vi "PRIOR_v.10.vi"() -> ()   [LabVIEW 2018]
uses:
  <vilib>/Instr/_visa.llb/VISA Configure Serial Port (Instr).vi
panel:
  in  "数字":i32
  in  "VISA resource name":refnum<visa-resource-name> caption="VISA资源名称"
  in  "返回Z轴坐标":bool
  in  "设置移动步长":bool
  in  "停止运动":bool
  out "error out":errorcluster
  out "读取缓冲区":string
  in  "error in (no error)":errorcluster caption="错误输入（无错误）"
  in  "down":bool
  in  "up":bool
  in  "停止":bool
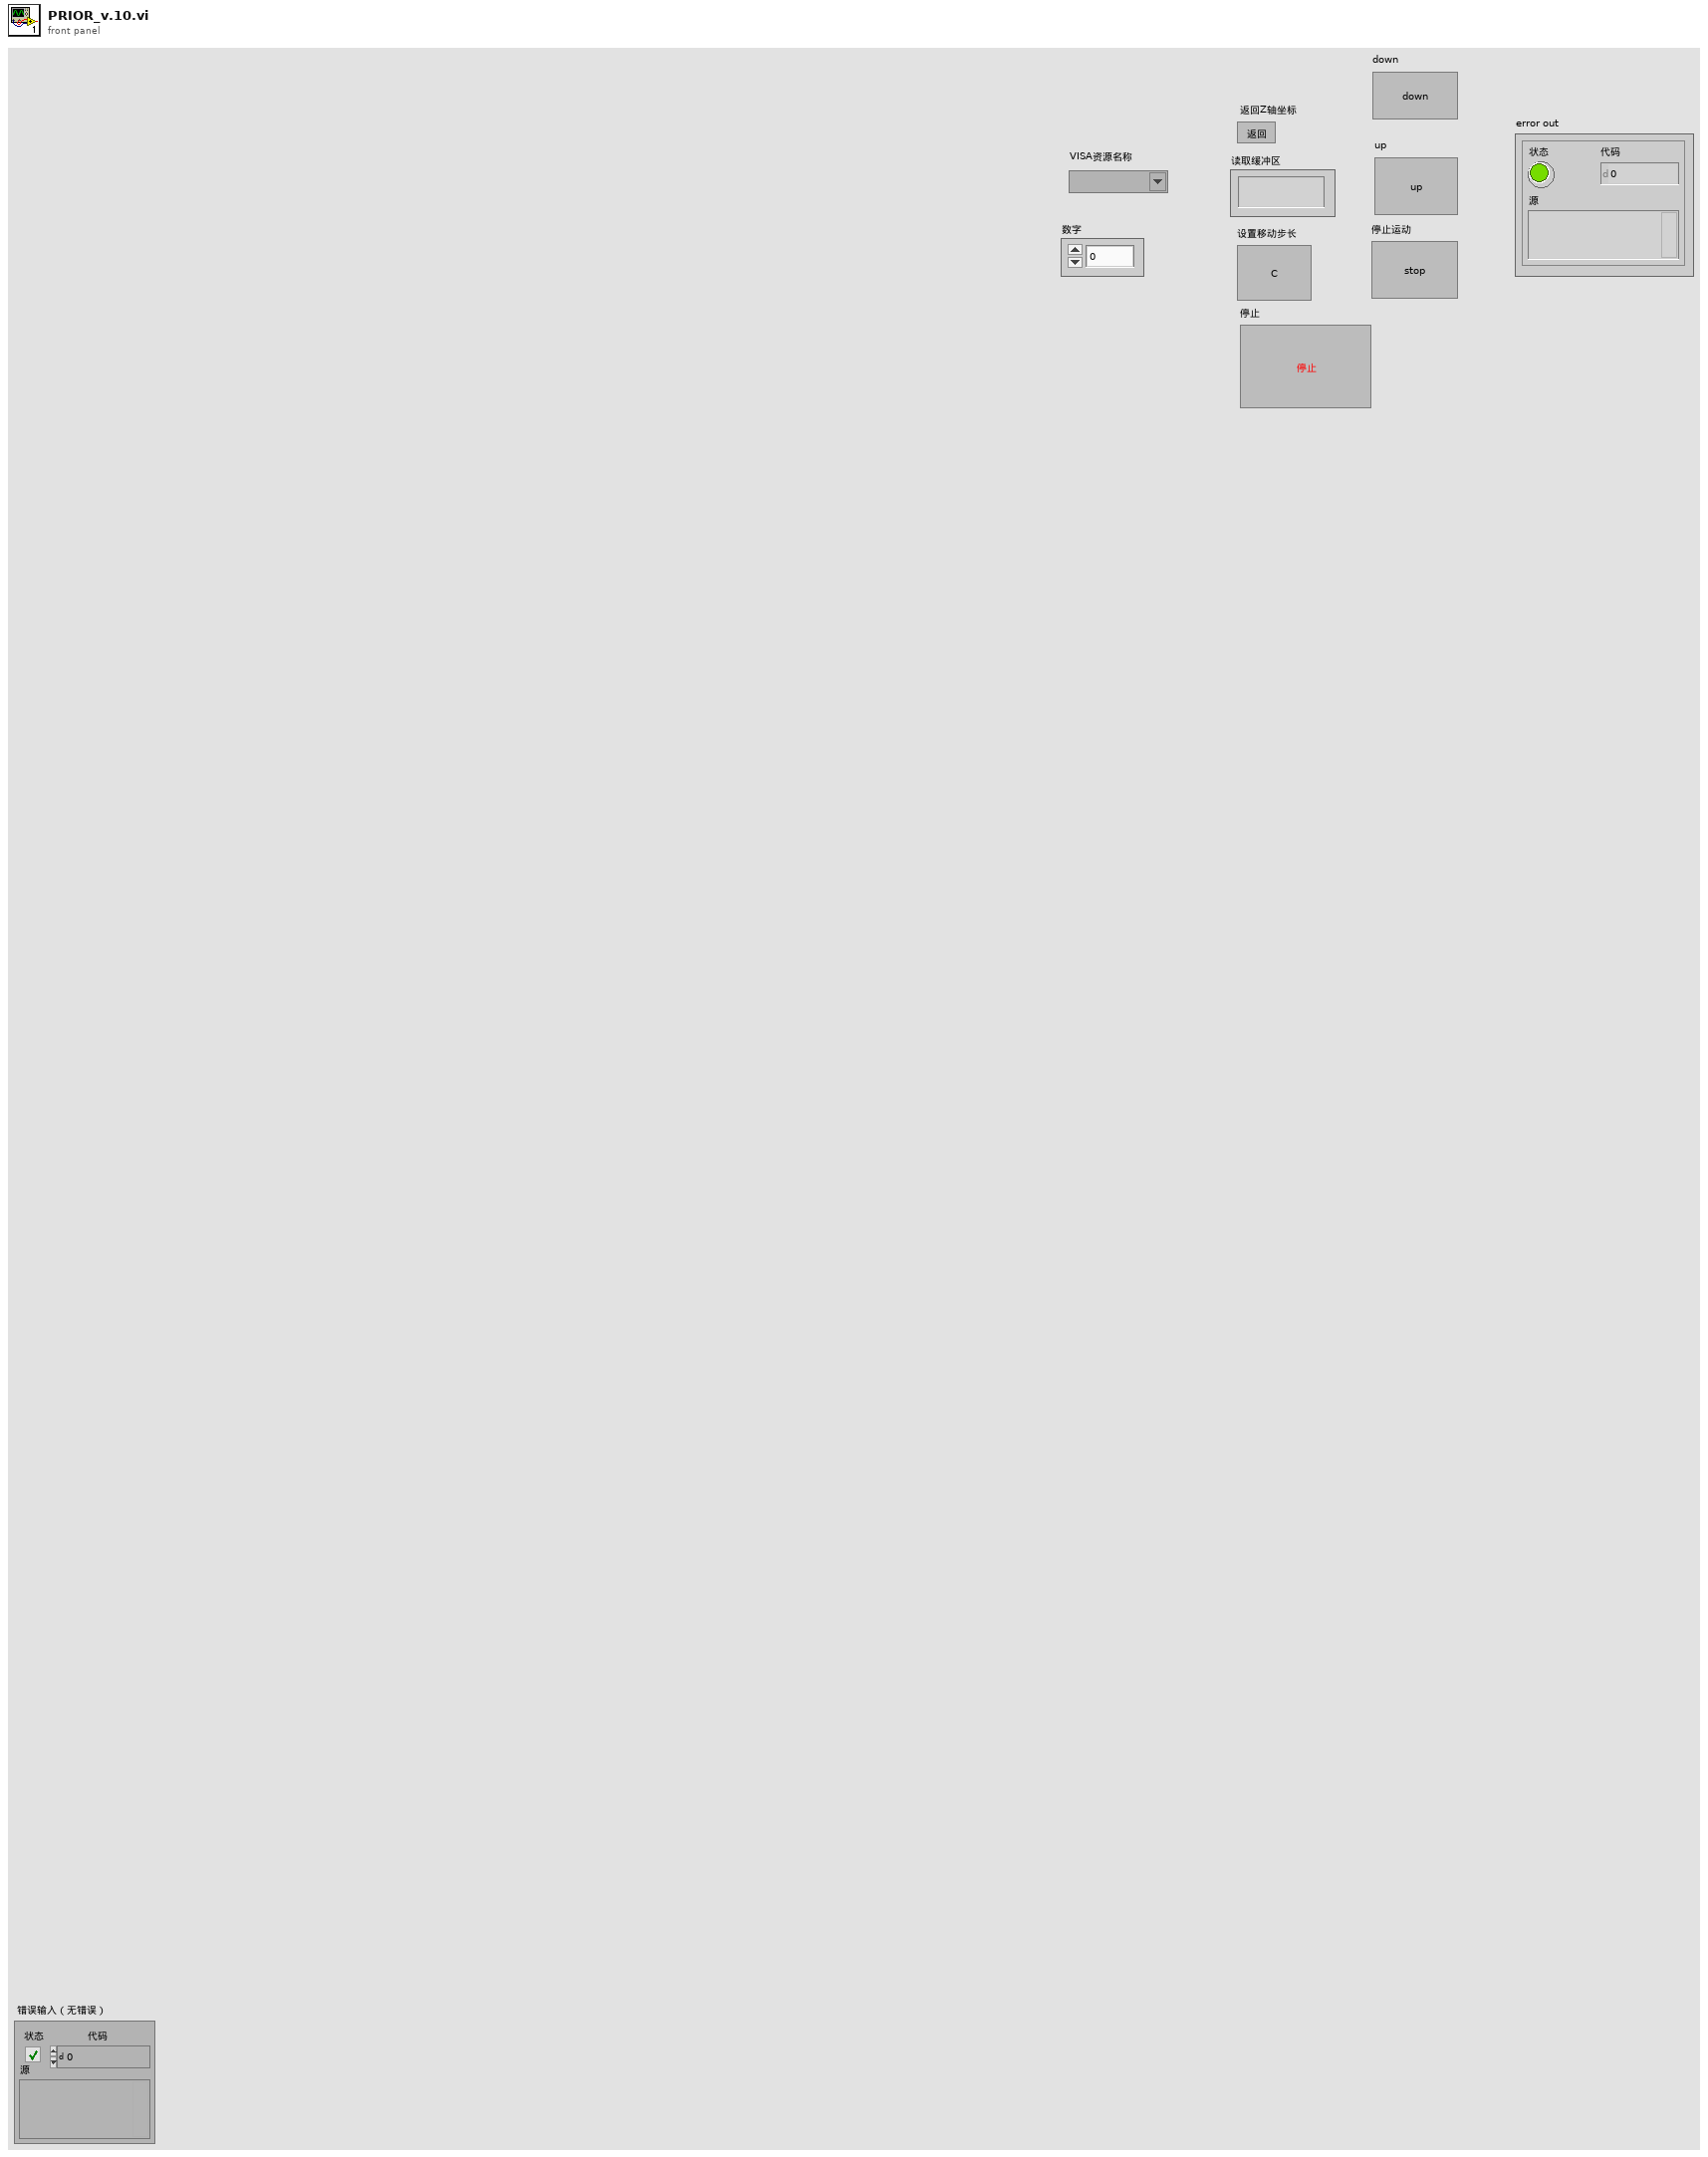
[diagram p1: front panel]
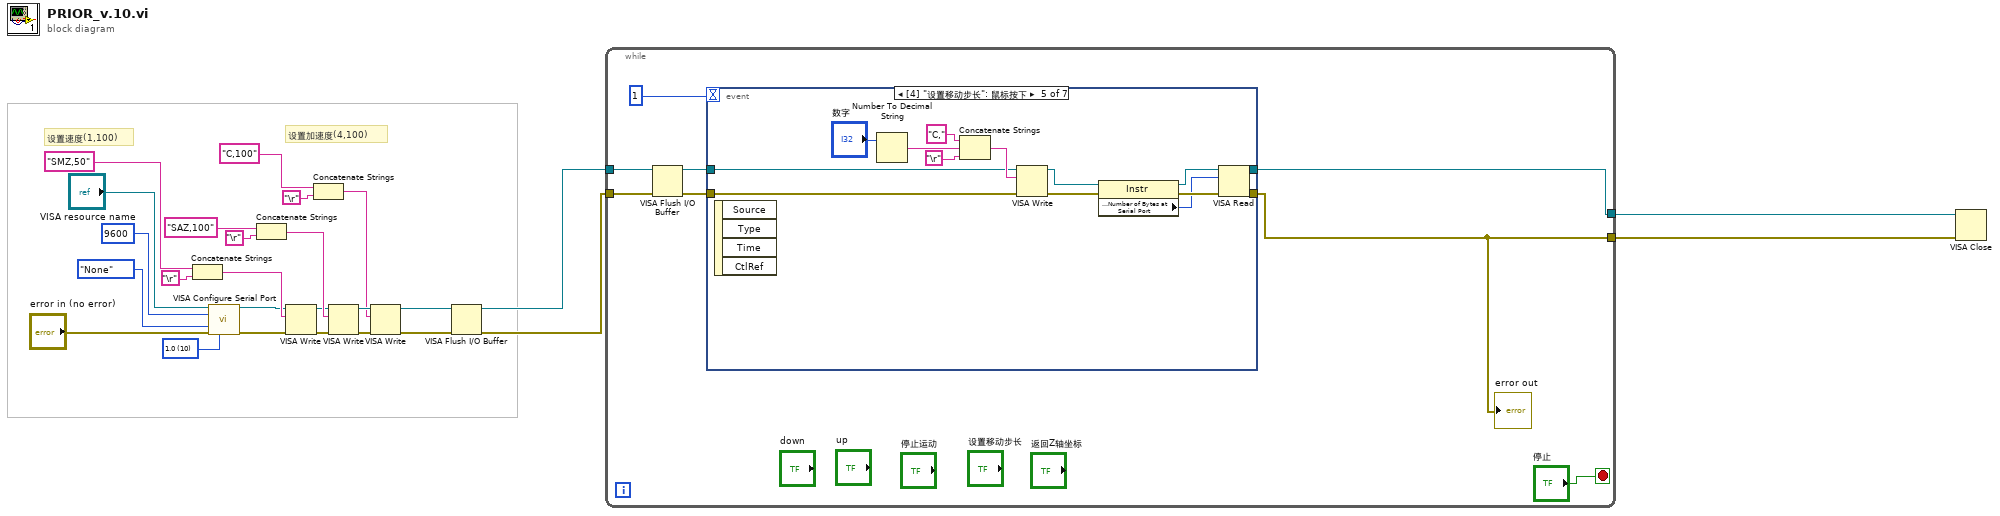
[diagram p0: block diagram]
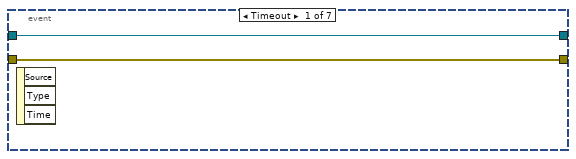
[diagram p2: hidden frame]
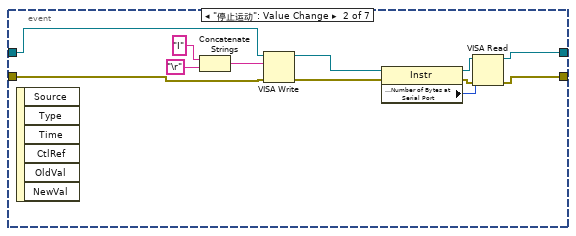
[diagram p3: hidden frame]
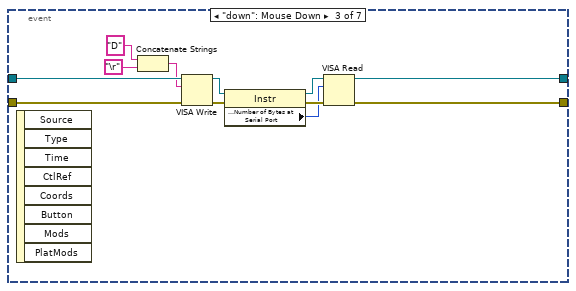
[diagram p4: hidden frame]
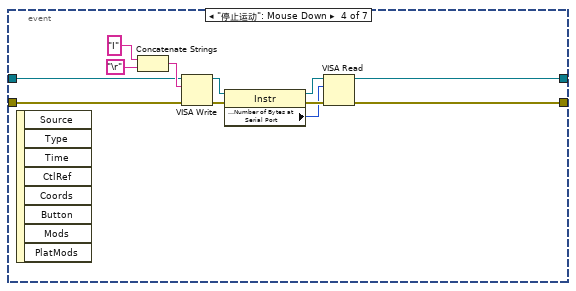
[diagram p5: hidden frame]
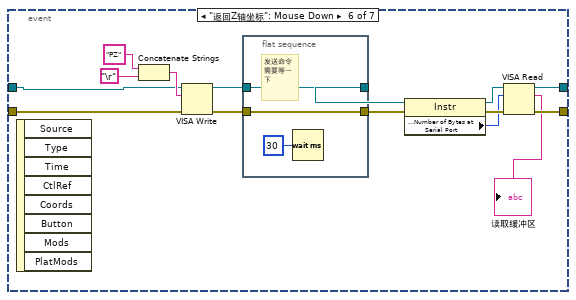
[diagram p6: hidden frame]
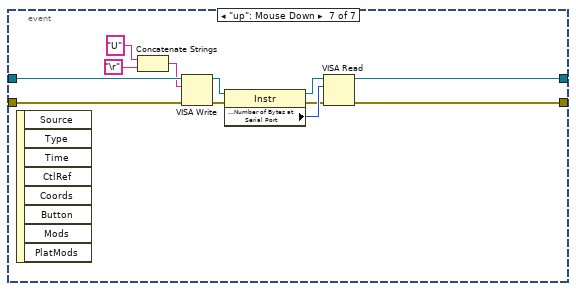
[diagram p7: hidden frame]
diagram:
  w24 = u16 10 items=["1.0"=10, "1.5"=15, "2.0"=20] ("停止位 (10: 1位)")
  # "设置加速度(4,100)"
  # "设置速度(1,100)"
  n1 = Concatenate Strings("SMZ,50" ("写入缓冲区"), "\r") -> (w20:string)
  n2 = call-poly "VISA Configure Serial Port"("VISA resource name"="VISA resource name", "baud rate (9600)"=u32 9600 ("波特率(9600)"), "parity (0:none)"=enum16{"None", "Odd", "Even", "Mark", "Space"}."None" ("校验（无）"), "error in (no error)"="error in (no error)", "stop bits (10: 1 bit)"=w24) -> ("VISA resource name out"=w18:refnum<visa-resource-name>, "error out"=w17:errorcluster)  [unwired: 9 in]
  n3 = Concatenate Strings("SAZ,100" ("写入缓冲区"), "\r") -> (w15:string)
  n4 = VISA Write ("VISA写入")(VISA resource name=w18, write buffer=w20, error in (no error)=w17) -> (VISA resource name out=w13:refnum<visa-resource-name>, error out=w12:errorcluster)  [unwired: 1 out]
  n5 = Concatenate Strings("C,100" ("写入缓冲区"), "\r") -> (w7:string)
  n6 = VISA Write ("VISA写入")(VISA resource name=w13, write buffer=w15, error in (no error)=w12) -> (VISA resource name out=w11:refnum<visa-resource-name>, error out=w10:errorcluster)  [unwired: 1 out]
  n7 = VISA Write ("VISA写入")(VISA resource name=w11, write buffer=w7, error in (no error)=w10) -> (VISA resource name out=w5:refnum<visa-resource-name>, error out=w4:errorcluster)  [unwired: 1 out]
  n8 = VISA Flush I/O Buffer(VISA resource name=w5, error in (no error)=w4) -> (VISA resource name out=w3:refnum<visa-resource-name>, error out=w2:errorcluster)  [unwired: 1 in]
  n9 = while {
    tunnel: w2 -> [w30]
    tunnel: w3 -> [w31]
    tunnel: [w27] -> w22
    tunnel: [w32] -> w6
    stop <- "停止" stop-if-true
    n10 = VISA Flush I/O Buffer(VISA resource name=w31, error in (no error)=w30) -> (VISA resource name out=w29:refnum<visa-resource-name>, error out=w28:errorcluster)  [unwired: 1 in]
    n11 = event shown="[4] \"设置移动步长\": 鼠标按下" {
      selector: _ -> [_ _ _ _ _ _ _]
      dyn-events: _ -> [_ _ _ _ _ _ _]
      timeout: 1 -> [_ _ _ _ _ _ _]
      tunnel: [w36 w38 w60 w62 w77 w93 w116] -> w32
      tunnel: [w35 w37 w59 w61 w76 w92 w115] -> w27
      tunnel: w29 -> [w36 w40 w58 w64 w79 w95 w114]
      tunnel: w28 -> [w35 w39 w57 w63 w78 w94 w113]
      event Timeout {
        n12 = event-data() -> ()  [unwired: 1 in, 3 out]
      }
      event "停止运动": Value Change {
        n13 = event-data() -> ()  [unwired: 1 in, 6 out]
        n14 = Concatenate Strings("I" ("写入缓冲区"), "\r") -> (w48:string)
        n15 = VISA Write ("VISA写入")(VISA resource name=w40, write buffer=w48, error in (no error)=w39) -> (VISA resource name out=w42:refnum<visa-resource-name>, error out=w41:errorcluster)  [unwired: 1 out]
        n16 = property class="Instr"(reference=w42, error in=w41) -> (reference out=w43:refnum<visa-resource-name>, error out=w44:errorcluster, "Serial Settings:Number of Bytes at Serial Port"=w45:u32)
        n17 = VISA Read(VISA resource name=w43, byte count=w45, error in (no error)=w44) -> (VISA resource name out=w38:refnum<visa-resource-name>, error out=w37:errorcluster)  [unwired: 2 out]
      }
      event "down": Mouse Down {
        n18 = event-data() -> ()  [unwired: 1 in, 8 out]
        n19 = Concatenate Strings("D" ("写入缓冲区"), "\r") -> (w49:string)
        n20 = VISA Write ("VISA写入")(VISA resource name=w58, write buffer=w49, error in (no error)=w57) -> (VISA resource name out=w55:refnum<visa-resource-name>, error out=w56:errorcluster)  [unwired: 1 out]
        n21 = property class="Instr"(reference=w55, error in=w56) -> (reference out=w54:refnum<visa-resource-name>, error out=w53:errorcluster, "Serial Settings:Number of Bytes at Serial Port"=w52:u32)
        n22 = VISA Read(VISA resource name=w54, byte count=w52, error in (no error)=w53) -> (VISA resource name out=w60:refnum<visa-resource-name>, error out=w59:errorcluster)  [unwired: 2 out]
      }
      event "停止运动": Mouse Down {
        n23 = event-data() -> ()  [unwired: 1 in, 8 out]
        n24 = Concatenate Strings("I" ("写入缓冲区"), "\r") -> (w65:string)
        n25 = VISA Write ("VISA写入")(VISA resource name=w64, write buffer=w65, error in (no error)=w63) -> (VISA resource name out=w71:refnum<visa-resource-name>, error out=w72:errorcluster)  [unwired: 1 out]
        n26 = property class="Instr"(reference=w71, error in=w72) -> (reference out=w70:refnum<visa-resource-name>, error out=w69:errorcluster, "Serial Settings:Number of Bytes at Serial Port"=w68:u32)
        n27 = VISA Read(VISA resource name=w70, byte count=w68, error in (no error)=w69) -> (VISA resource name out=w62:refnum<visa-resource-name>, error out=w61:errorcluster)  [unwired: 2 out]
      }
      event "设置移动步长": Mouse Down {
        n28 = event-data() -> ()  [unwired: 1 in, 4 out]
        n29 = Number To Decimal String(number="数字") -> (decimal integer string=w74:string)  [unwired: 1 in]
        n30 = Concatenate Strings("C," ("写入缓冲区"), w74, "\r") -> (w80:string)
        n31 = VISA Write ("VISA写入")(VISA resource name=w79, write buffer=w80, error in (no error)=w78) -> (VISA resource name out=w85:refnum<visa-resource-name>, error out=w86:errorcluster)  [unwired: 1 out]
        n32 = property class="Instr"(reference=w85, error in=w86) -> (reference out=w84:refnum<visa-resource-name>, error out=w83:errorcluster, "Serial Settings:Number of Bytes at Serial Port"=w82:u32)
        n33 = VISA Read(VISA resource name=w84, byte count=w82, error in (no error)=w83) -> (VISA resource name out=w77:refnum<visa-resource-name>, error out=w76:errorcluster)  [unwired: 2 out]
      }
      event "返回Z轴坐标": Mouse Down {
        n34 = event-data() -> ()  [unwired: 1 in, 8 out]
        n35 = Concatenate Strings("PZ" ("写入缓冲区"), "\r") -> (w97:string)
        n36 = VISA Write ("VISA写入")(VISA resource name=w95, write buffer=w97, error in (no error)=w94) -> (VISA resource name out=w91:refnum<visa-resource-name>, error out=w90:errorcluster)  [unwired: 1 out]
        n37 = flat-sequence {
          tunnel: w91 -> [w103]
          tunnel: w90 -> [w104]
          tunnel: [w104] -> w88
          tunnel: [w103] -> w89
          frame #0 {
            # "发送命令需要等一下"
            n38 = Wait (ms)(milliseconds to wait=u32 30 ("等待时间（毫秒）")) -> ()  [unwired: 1 out]
          }
        }
        n39 = property class="Instr"(reference=w89, error in=w88) -> (reference out=w101:refnum<visa-resource-name>, error out=w100:errorcluster, "Serial Settings:Number of Bytes at Serial Port"=w99:u32)
        n40 = VISA Read(VISA resource name=w101, byte count=w99, error in (no error)=w100) -> (VISA resource name out=w93:refnum<visa-resource-name>, read buffer=→"读取缓冲区":string, error out=w92:errorcluster)  [unwired: 1 out]
      }
      event "up": Mouse Down {
        n41 = event-data() -> ()  [unwired: 1 in, 8 out]
        n42 = Concatenate Strings("U" ("写入缓冲区"), "\r") -> (w110:string)
        n43 = VISA Write ("VISA写入")(VISA resource name=w114, write buffer=w110, error in (no error)=w113) -> (VISA resource name out=w109:refnum<visa-resource-name>, error out=w108:errorcluster)  [unwired: 1 out]
        n44 = property class="Instr"(reference=w109, error in=w108) -> (reference out=w106:refnum<visa-resource-name>, error out=w105:errorcluster, "Serial Settings:Number of Bytes at Serial Port"=w107:u32)
        n45 = VISA Read(VISA resource name=w106, byte count=w107, error in (no error)=w105) -> (VISA resource name out=w116:refnum<visa-resource-name>, error out=w115:errorcluster)  [unwired: 2 out]
      }
    }
    "error out" <- w27
  }
  n46 = VISA Close(VISA resource name=w6, error in (no error)=w22) -> ()  [unwired: 1 out]
